vi "countSteps.vi"(3 "direction":i32, 4 "axis":i32, 5 "errorIn":errorcluster, 6 "referenceIn":refnum<k24>) -> (0 "nSteps":i32, 1 "error_out":errorcluster, 2 "referenceOut":refnum<k24>)   [LabVIEW 2020]
uses:
  C:/Program Files/Newport/Piezo Motion Control/Newport AG-UC2-UC8 Applet/Samples/LabVIEW 2009/AgilisCmdLib.dll
  Program Files/Newport/Piezo Motion Control/Newport AG-UC2-UC8 Applet/Samples/LabVIEW 2009/AgilisCmdLib.dll
panel:
  # "This VI requires the device to be at a limit."
  # "Parameter \"direction\" must be either +1 (pos. direction) or -1 (neg. direction)."
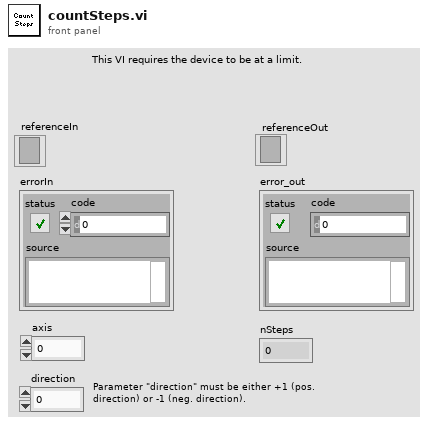
[diagram p1: front panel]
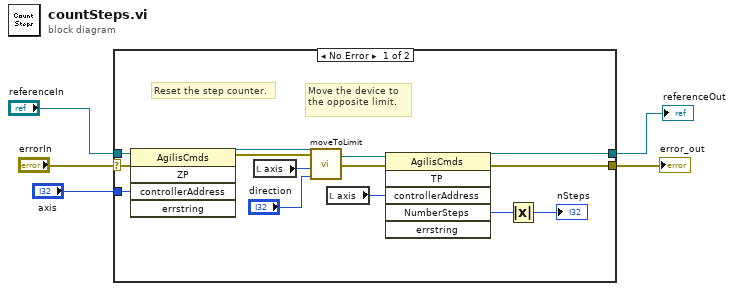
[diagram p0: block diagram]
diagram:
  n1 = case shown="No Error" "errorIn" {
    selector: "errorIn" -> [w8 w20]
    tunnel: "referenceIn" -> [w19 w21]
    tunnel: "axis" -> [w18 _]
    tunnel: [w10 w21] -> w3
    tunnel: [w9 w20] -> w2
    frame No Error {
      # "Move the device to the opposite limit."
      # "Reset the step counter."
      n2 = invoke class="AgilisCmds" method="ZP"(reference=w19, error in=w8, "controllerAddress"=w18) -> (reference out=w17:refnum<k24>, error out=w16:errorcluster)  [unwired: 2 in, 3 out]
      n3 = local read "axis"() -> (w15:i32)
      n4 = call "moveToLimit.vi"("direction"="direction", "axis"=w15, "errorIn"=w16, "referenceIn"=w17) -> ("errorOut"=w12:errorcluster, "referenceOut"=w13:refnum<k24>)
      n5 = local read "axis"() -> (w11:i32)
      n6 = invoke class="AgilisCmds" method="TP"(reference=w13, error in=w12, "controllerAddress"=w11) -> (reference out=w10:refnum<k24>, error out=w9:errorcluster, "NumberSteps"=w7:i32)  [unwired: 3 in, 3 out]
      n7 = Absolute Value(x=w7) -> (abs(x)=→"nSteps":i32)
    }
    frame Error {
    }
  }
  "referenceOut" <- w3
  "error_out" <- w2
